vi "Update Referenced Nodes TypeName.vi"(8 "error in":errorcluster, 9 "New TypeName":string, 11 "Old TypeName":string) -> (0 "error out":errorcluster)   [LabVIEW 2025]
uses:
  Types/TD NodeRef Map Action.ctl
  <resource>/objmgr/DOMUserDefRef.rc
  Types/CD NodeRef Map Action.ctl
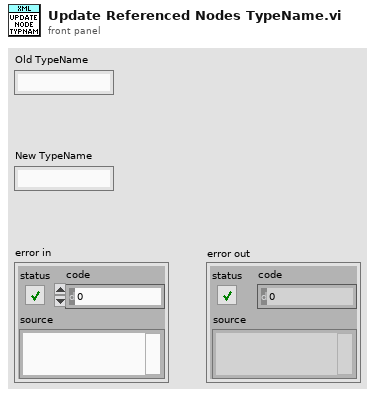
[diagram p1: front panel]
types:
  T1 = typedef "CD NodeRef Map Action.ctl" = enum16{"Init", "Add XMLNodeRef", "Update ParentName", "Delete XMLNodeRef", "Get All Keys", "Get", "skip"}
  T2 = typedef "TD NodeRef Map Action.ctl" = enum16{"Init", "Add XMLNodeRef", "Delete XMLNodeRef", "Add TDNodeRefs", "Delete TDNodeRefs", "Clear TDNodeRefs", "Add ChildXMLNodeRef", "Delete ChildXMLNodeRef", "Get All Keys", "Update ParentName", "Get", "skip"}
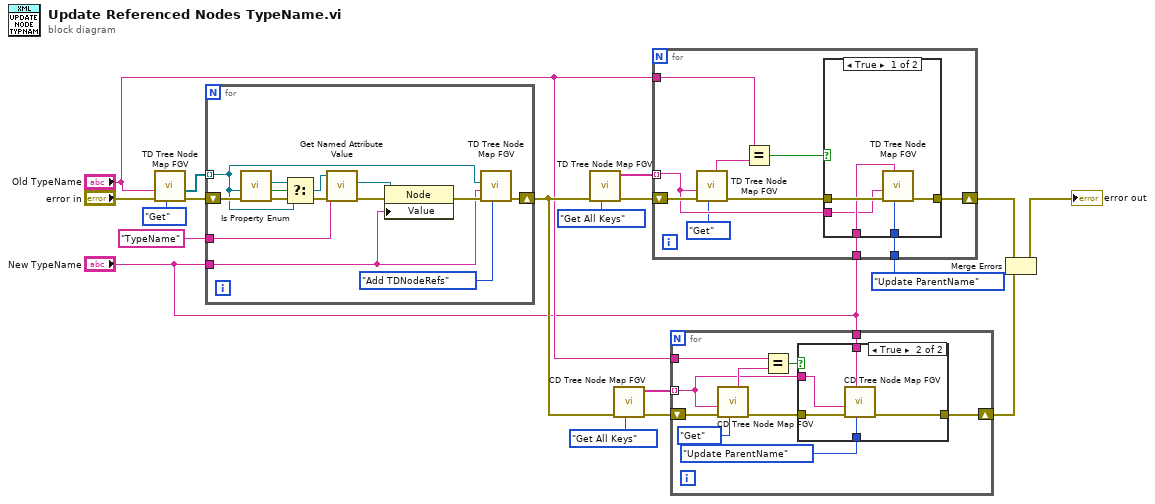
[diagram p0: block diagram]
diagram:
  n1 = call "TD Tree Node Map FGV.vi"("Action"=TD_NodeRef_Map_Action."Get", "error in"="error in", "Node Name"="Old TypeName") -> ("error out"=w16:errorcluster, "ReferencedNodes"=w13:refnum<k20>[])  [unwired: 3 in, 4 out]
  n2 = for {
    tunnel: w13 -> [w19] mode=indexing
    shift-right: [w27] -> w9
    shift-left: w16 -> [w25]
    tunnel: "TypeName" ("Attribute Name") -> [w23]
    tunnel: "New TypeName" -> [w28]
    n3 = call "Is Property Enum.vi"("error in"=w25, "Node"=w19) -> ("error out"=w24:errorcluster, "Is Enum Property"=w22:bool, "Enum Node"=w20:refnum<k20>)  [unwired: 7 in]
    n4 = Select(t=w20, s=w22, f=w19) -> (s? t:f=w21:refnum<k20>)
    n5 = call "Get Named Attribute Value.vi"("error in"=w24, "Attribute Name"=w23, "Node In"=w21) -> ("error out"=w31:errorcluster, "Attribute Node"=w30:refnum<k20>)  [unwired: 5 in, 2 out]
    n6 = property class="Node"(reference=w30, error in=w31, "Value"=w28) -> (error out=w29:errorcluster)  [unwired: 1 out]
    n7 = call "TD Tree Node Map FGV.vi"("Action"=TD_NodeRef_Map_Action."Add TDNodeRefs", "error in"=w29, "Node Name"=w28, "Attribute Node"=w19) -> ("error out"=w27:errorcluster)  [unwired: 2 in, 5 out]
  }
  n8 = call "TD Tree Node Map FGV.vi"("Action"=TD_NodeRef_Map_Action."Get All Keys", "error in"=w9) -> ("error out"=w10:errorcluster, "All Node Names"=w11:string[])  [unwired: 4 in, 4 out]
  n9 = call "CD Tree Node Map FGV.vi"("Action"=CD_NodeRef_Map_Action."Get All Keys", "error in"=w9) -> ("error out"=w6:errorcluster, "Map Keys"=w7:string[])  [unwired: 5 in, 3 out]
  n10 = for {
    shift-right: [w41] -> w2
    shift-left: w10 -> [w38]
    tunnel: TD_NodeRef_Map_Action."Update ParentName" ("Action") -> [w40]
    tunnel: "New TypeName" -> [w39]
    tunnel: w11 -> [w33] mode=indexing
    tunnel: "Old TypeName" -> [w35]
    n11 = call "TD Tree Node Map FGV.vi"("Action"=TD_NodeRef_Map_Action."Get", "error in"=w38, "Node Name"=w33) -> ("error out"=w37:errorcluster, "Parent Node out"=w36:string)  [unwired: 3 in, 4 out]
    n12 = Equal?(x=w35, y=w36) -> (x = y?=w34:bool)
    n13 = case shown="True" w34 {
      tunnel: w37 -> [w46 w47]
      tunnel: [w45 w47] -> w41
      tunnel: w40 -> [w44 _]
      tunnel: w39 -> [w43 _]
      tunnel: w33 -> [w42 _]
      frame True {
        n14 = call "TD Tree Node Map FGV.vi"("Action"=w44, "Parent Node"=w43, "error in"=w46, "Node Name"=w42) -> ("error out"=w45:errorcluster)  [unwired: 2 in, 5 out]
      }
      frame False {
      }
    }
  }
  n15 = for {
    tunnel: w7 -> [w51] mode=indexing
    shift-right: [w48] -> w3
    shift-left: w6 -> [w57]
    tunnel: "Old TypeName" -> [w54]
    tunnel: "New TypeName" -> [w50]
    n16 = call "CD Tree Node Map FGV.vi"("Action"=CD_NodeRef_Map_Action."Get", "error in"=w57, "Node Name"=w51) -> ("error out"=w52:errorcluster, "Parent Name out"=w55:string)  [unwired: 4 in, 3 out]
    n17 = Equal?(x=w54, y=w55) -> (x = y?=w53:bool)
    n18 = case shown="True" w53 {
      tunnel: w52 -> [w58 w63]
      tunnel: w51 -> [_ w62]
      tunnel: w50 -> [_ w61]
      tunnel: CD_NodeRef_Map_Action."Update ParentName" ("Action") -> [_ w60]
      tunnel: [w58 w59] -> w48
      frame False {
      }
      frame True {
        n19 = call "CD Tree Node Map FGV.vi"("Action"=w60, "Parent Name in"=w61, "error in"=w63, "Node Name"=w62) -> ("error out"=w59:errorcluster)  [unwired: 3 in, 4 out]
      }
    }
  }
  n20 = Merge Errors(w2, w3) -> (→"error out":errorcluster)
